vi "Create Data Channels.vi"(8 "error in":errorcluster, 11 "Node In":refnum<class "AMS Climate Chamber Template.lvclass">) -> (0 "error out":errorcluster, 3 "Node Out":refnum<class "AMS Climate Chamber Template.lvclass">)   [LabVIEW 2023, in "AMS Climate Chamber Template.lvlib" / "AMS Climate Chamber Template.lvclass"]
uses:
  AMS Climate Chamber Template.lvclass
  C:/Program Files/National Instruments/LabVIEW 2024/vi.lib/ADAS Replay HIL/Template Node/Plugin/Template Node/Template Node.lvclass
  <vilib>/ADAS Replay HIL/Template Node/Plugin/Template Node/Template Node.lvclass/Template Node.ctl
  AMS Climate Chamber Template.lvclass/AMS Climate Chamber Template.ctl
  C:/Program Files/National Instruments/AMS plugin/Capabilities/Capabilities/High Level Capabilities/Climate Chamber/Climate Chamber.lvclass
  <vilib>/ADAS Replay HIL/Template Node/Plugin/Template Node/Template Node.lvclass
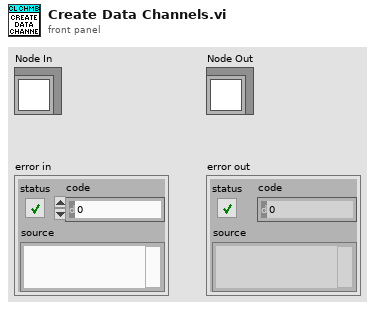
[diagram p1: front panel]
types:
  T1 = typedef "AMS Climate Chamber Template.lvlib/AMS Climate Chamber Template.lvclass/Configuration Params.ctl" = cluster{"Common":T2, "Amount of Channels":u32, "Address":string}
  T2 = typedef "Template Node.lvlib/Template Node.lvclass/Common Configuration Params.ctl" = cluster{"Iteration Interval (s)":dbl, "T0 (ns)":u64, "Priority":i32, "Processor":i32, "Wait in Ready State":bool}
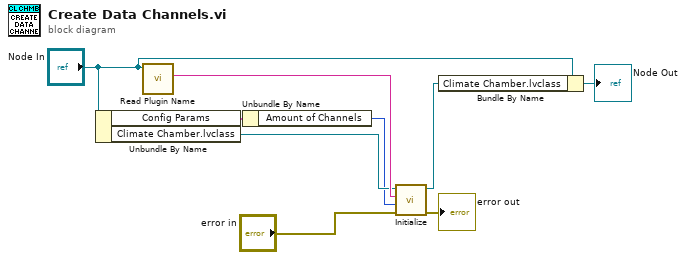
[diagram p0: block diagram]
diagram:
  n1 = Unbundle By Name("Node In") -> ("Config Params"=w6:T1, "Climate Chamber.lvclass"=w7:refnum<class "Climate Chamber.lvclass">)
  n2 = call <vilib>:"Read Plugin Name.vi"("Template Node in"="Node In") -> ("Plugin Name"=w9:string)  [unwired: 8 in, 2 out]
  n3 = Unbundle By Name(w6) -> ("Amount of Channels"=w5:u32)
  n4 = call-dynamic "Initialize.vi"("error in"="error in", "Number of Channels"=w5, "Instance Name"=w9, "Climate Chamber in"=w7) -> ("error out"=→"error out":errorcluster, "Climate Chamber out"=w8:refnum<class "Climate Chamber.lvclass">)  [unwired: 5 in, 1 out]
  n5 = Bundle By Name(cluster="Node In", "Climate Chamber.lvclass"=w8) -> (→"Node Out":refnum<class "AMS Climate Chamber Template.lvclass">)
